vi "Main.vi"() -> ()   [LabVIEW 2017]
uses:
  <vilib>/Utility/error.llb/DialogType.ctl
  <vilib>/Instr/_visa.llb/VISA Configure Serial Port (Serial Instr).vi
panel:
  in  "RUN":bool
  out "Error Messages":string
  in  "Path":path
  in  "Port 2":refnum<visa-resource-name>
  in  "Port 1":refnum<visa-resource-name>
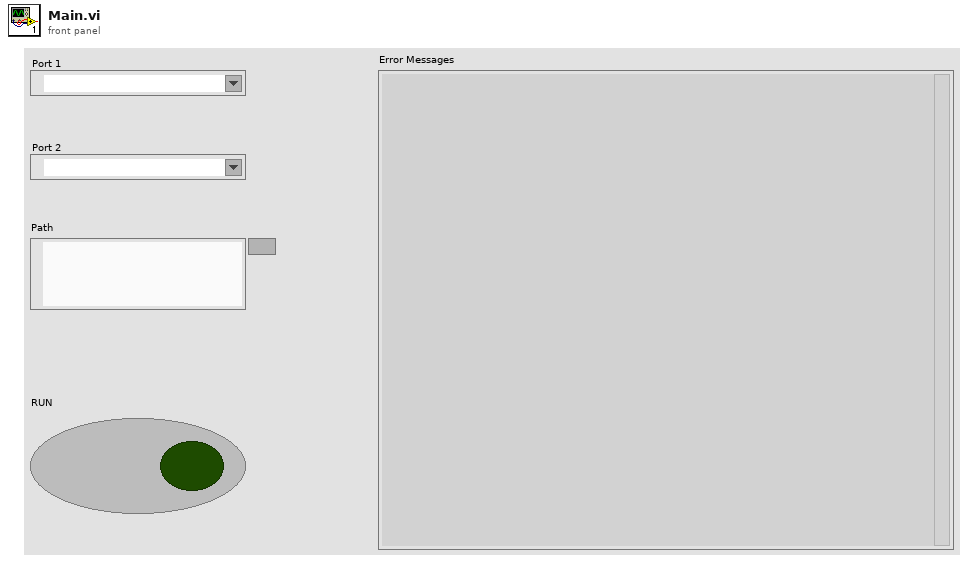
[diagram p1: front panel]
types:
  T1 = cluster{"Port":i8, "Time":timestamp, "Message":string}
  T2 = enum16{"open", "replace", "create", "open or create", "replace or create", "replace or create with confirmation"}
  T3 = typedef "LVDateTimeRec.ctl" = cluster{"fractional second":dbl, "second":i32, "minute":i32, "hour":i32, "day of month":i32, "month":i32, "year":i32, "day of week":i32, "day of year":i32, "DST":i32}
  T4 = typedef "DialogType.ctl" = u16
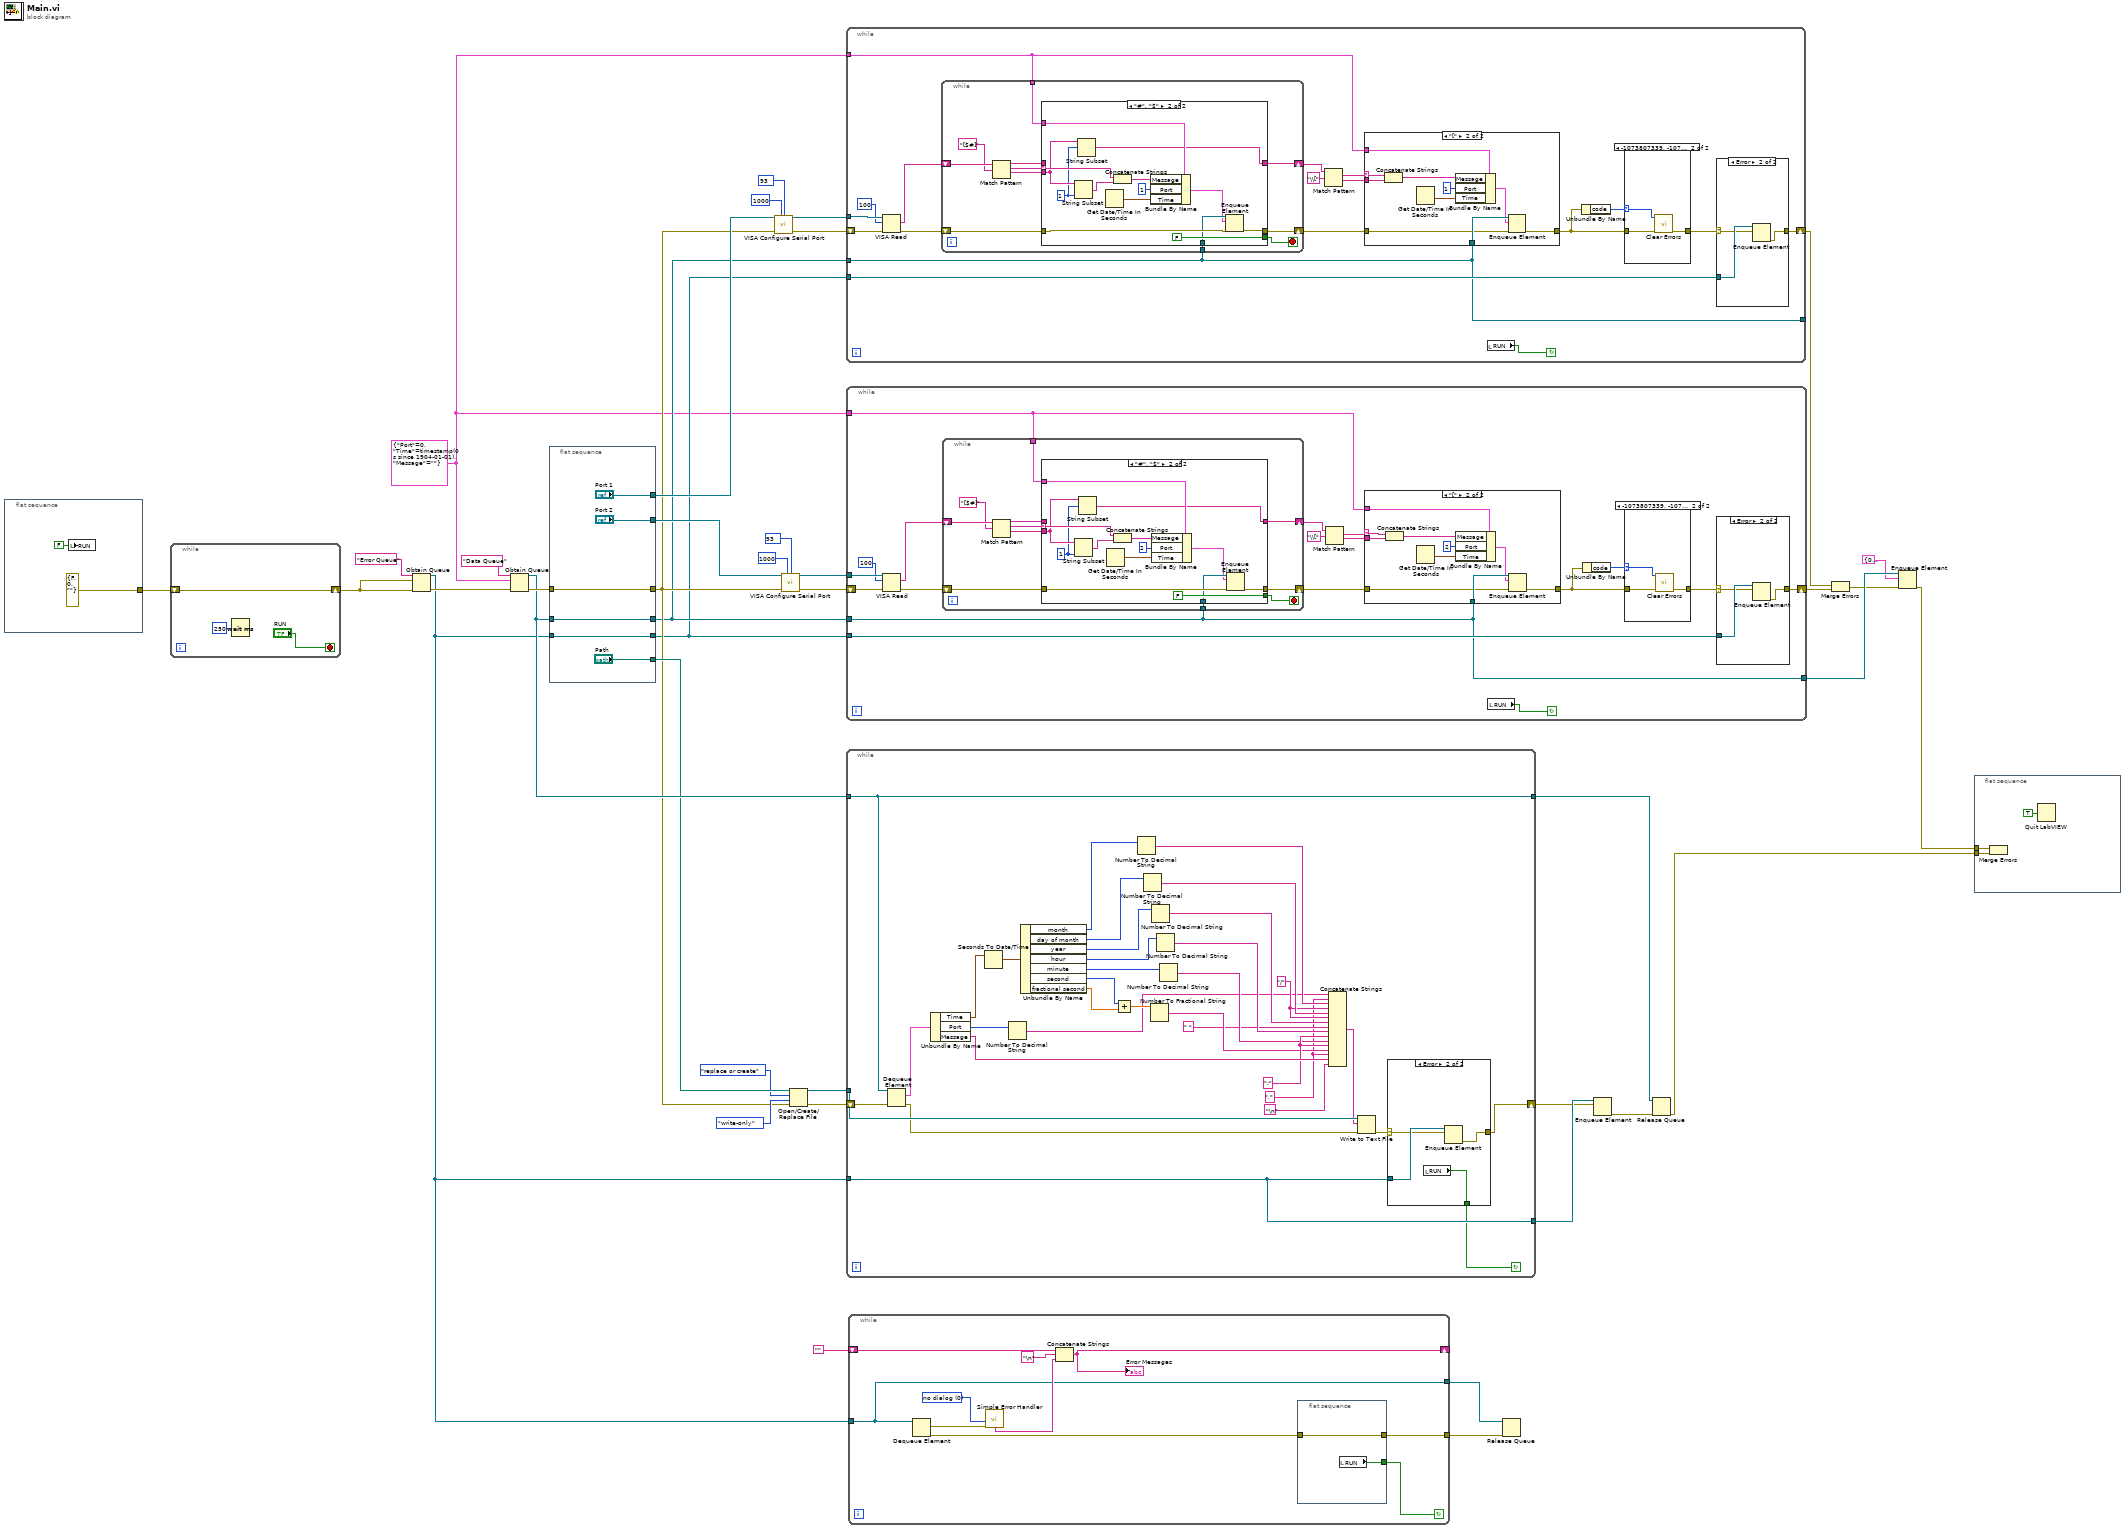
[diagram p0: block diagram]
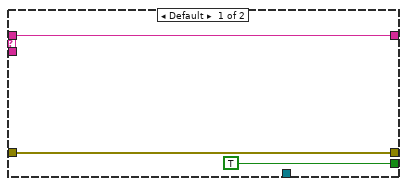
[diagram p2: hidden frame]
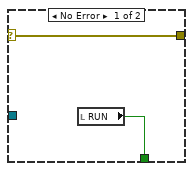
[diagram p6: hidden frame]
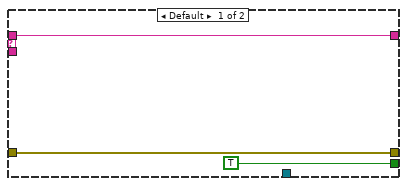
[diagram p7: hidden frame]
diagram:
  w7 = T1 {"Port"=0, "Time"=timestamp(0 s since 1904-01-01), "Message"=""}
  n1 = flat-sequence {
    tunnel: [errorcluster {"status"=FALSE, "code"=0, "source"=""} ("error constant")] -> w41
    frame #0 {
      n2 = local write "RUN"(FALSE ("RUN")) -> ()
    }
  }
  n3 = while {
    shift-right: [w46] -> w40
    shift-left: w41 -> [w46]
    stop <- "RUN" stop-if-true
    n4 = Wait (ms)(milliseconds to wait=u32 250) -> ()  [unwired: 1 out]
  }
  n5 = Obtain Queue(name (unnamed)="Error Queue", element data type=w40, error in (no error)=w40) -> (queue out=w20:refnum<queue>, error out=w38:errorcluster)  [unwired: 2 in, 1 out]
  n6 = Obtain Queue(name (unnamed)="Data Queue", element data type=w7, error in (no error)=w38) -> (queue out=w31:refnum<queue>, error out=w36:errorcluster)  [unwired: 2 in, 1 out]
  n7 = flat-sequence {
    tunnel: w31 -> [w52]
    tunnel: w36 -> [w51]
    tunnel: w20 -> [w50]
    tunnel: [w52] -> w9
    tunnel: [w51] -> w10
    tunnel: [w50] -> w8
    tunnel: ["Port 1"] -> w11
    tunnel: ["Port 2"] -> w12
    tunnel: ["Path"] -> w29
    frame #0 {
    }
  }
  n8 = call-poly "VISA Configure Serial Port"("VISA resource name"=w11, "timeout (10sec)"=u32 1000, "termination char\n(0xA = '\\n' = LF)"=u8 93 ("termination char\n(0xA = '\\n' = LF)"), "error in (no error)"=w10) -> ("VISA resource name out"=w14:refnum<visa-resource-name>, "error out"=w13:errorcluster)  [unwired: 10 in]
  n9 = call-poly "VISA Configure Serial Port"("VISA resource name"=w12, "timeout (10sec)"=u32 1000, "termination char\n(0xA = '\\n' = LF)"=u8 93 ("termination char\n(0xA = '\\n' = LF)"), "error in (no error)"=w10) -> ("VISA resource name out"=w33:refnum<visa-resource-name>, "error out"=w32:errorcluster)  [unwired: 10 in]
  n10 = Open/Create/Replace File(file path (use dialog)=w29, error in=w10, operation (0:open)=T2."replace or create", access (0:read/write)=enum16{"read/write", "read-only", "write-only"}."write-only") -> (refnum out=w30:refnum<file>, error out=w26:errorcluster)  [unwired: 2 in, 1 out]
  n11 = while {
    tunnel: w14 -> [w70]
    tunnel: w7 -> [w55]
    tunnel: w9 -> [w54]
    tunnel: w8 -> [w65]
    shift-right: [w64] -> w5
    shift-left: w13 -> [w69]
    tunnel: [w54] -> _
    stop <- w63 continue-if-true
    n12 = VISA Read(VISA resource name=w70, byte count=u32 100, error in (no error)=w69) -> (read buffer=w58:string, error out=w56:errorcluster)  [unwired: 2 out]
    n13 = while {
      shift-right: [w75] -> w57
      shift-left: w58 -> [w81]
      shift-right: [w74] -> w53
      shift-left: w56 -> [w76]
      tunnel: w55 -> [w72]
      tunnel: w54 -> [w71]
      stop <- w73 stop-if-true
      n14 = Match Pattern(string=w81, regular expression="[$#]") -> (before substring=w78:string, match substring=w79:string, after substring=w77:string)  [unwired: 1 in, 1 out]
      n15 = case shown="\"#\", \"$\"" w79 {
        selector: w79 -> [_ w97]
        tunnel: w78 -> [w84 _]
        tunnel: w77 -> [_ w89]
        tunnel: w76 -> [w83 w94]
        tunnel: [w84 w87] -> w75
        tunnel: [w83 w95] -> w74
        tunnel: [TRUE FALSE] -> w73
        tunnel: w72 -> [_ w92]
        tunnel: w71 -> [_ w93]
        frame Default {
        }
        frame "#", "$" {
          w88 = 1 ("length (rest)")
          n16 = String Subset(string=w89, length (rest)=w88) -> (substring=w96:string)  [unwired: 1 in]
          n17 = String Subset(string=w89, offset (0)=w88) -> (substring=w87:string)  [unwired: 1 in]
          n18 = Get Date/Time In Seconds() -> (seconds since 1Jan1904=w85:timestamp)
          n19 = Concatenate Strings(w97, w96) -> (w90:string)
          n20 = Bundle By Name(cluster=w92, "Message"=w90, "Port"=i8 1, "Time"=w85) -> (w91:T1)
          n21 = Enqueue Element(queue=w93, element=w91, error in (no error)=w94) -> (error out=w95:errorcluster)  [unwired: 1 in, 2 out]
        }
      }
    }
    n22 = Match Pattern(string=w57, regular expression="\\[") -> (match substring=w67:string, after substring=w66:string)  [unwired: 1 in, 2 out]
    n23 = case shown="\"[\"" w67 {
      selector: w67 -> [_ w116]
      tunnel: w66 -> [_ w117]
      tunnel: w55 -> [_ w115]
      tunnel: w53 -> [w107 w110]
      tunnel: w54 -> [_ w111]
      tunnel: [w107 w108] -> w59
      frame Default {
      }
      frame "[" {
        n24 = Concatenate Strings(w116, w117) -> (w114:string)
        n25 = Get Date/Time In Seconds() -> (seconds since 1Jan1904=w112:timestamp)
        n26 = Bundle By Name(cluster=w115, "Message"=w114, "Port"=i8 1, "Time"=w112) -> (w109:T1)
        n27 = Enqueue Element(queue=w111, element=w109, error in (no error)=w110) -> (error out=w108:errorcluster)  [unwired: 1 in, 2 out]
      }
    }
    n28 = local read "RUN"() -> (w63:bool)
    n29 = Unbundle By Name(w59) -> ("code"=w61:i32)
    n30 = case shown="-1073807339, -1073807298, -1073807253" w61 {
      selector: w61 -> [_ w102]
      tunnel: [w99 w100] -> w60
      tunnel: w59 -> [w99 w101]
      frame Default {
      }
      frame -1073807339, -1073807298, -1073807253 {
        n31 = call <vilib>:"Clear Errors.vi"("error in (no error)"=w101, "specific error code to clear (0: all)"=w102) -> ("error out"=w100:errorcluster)  [unwired: 4 in, 1 out]
      }
    }
    n32 = case shown="Error" w60 {
      selector: w60 -> [w103 w105]
      tunnel: w65 -> [_ w106]
      tunnel: [w103 w104] -> w64
      frame No Error {
      }
      frame Error {
        n33 = Enqueue Element(queue=w106, element=w105) -> (error out=w104:errorcluster)  [unwired: 2 in, 2 out]
      }
    }
  }
  n34 = while {
    tunnel: w31 -> [w140]
    tunnel: w30 -> [w146]
    tunnel: w20 -> [w141]
    shift-right: [w142] -> w3
    shift-left: w26 -> [w151]
    tunnel: [w141] -> w23
    tunnel: [w140] -> w21
    stop <- w139 continue-if-true
    w120 = "/" ("string")
    w133 = ":" ("string")
    w119 = "," ("string")
    n35 = Dequeue Element(queue=w140, error in (no error)=w151) -> (element=w150:T1, error out=w144:errorcluster)  [unwired: 1 in, 2 out]
    n36 = Unbundle By Name(w150) -> ("Time"=w138:timestamp, "Port"=w149:i8, "Message"=w148:string)
    n37 = Seconds To Date/Time(time stamp (now)=w138) -> (date time rec=w137:T3)  [unwired: 1 in]
    n38 = Number To Decimal String(number=w149) -> (decimal integer string=w118:string)  [unwired: 1 in]
    n39 = Unbundle By Name(w137) -> ("month"=w125:i32, "day of month"=w126:i32, "year"=w127:i32, "hour"=w128:i32, "minute"=w136:i32, "second"=w134:i32, "fractional second"=w135:dbl)
    n40 = Add(x=w134, y=w135) -> (x+y=w130:dbl)
    n41 = Number To Decimal String(number=w125) -> (decimal integer string=w122:string)  [unwired: 1 in]
    n42 = Number To Decimal String(number=w126) -> (decimal integer string=w123:string)  [unwired: 1 in]
    n43 = Number To Fractional String(number=w130) -> (F-format string=w129:string)  [unwired: 3 in]
    n44 = Number To Decimal String(number=w127) -> (decimal integer string=w124:string)  [unwired: 1 in]
    n45 = Number To Decimal String(number=w128) -> (decimal integer string=w132:string)  [unwired: 1 in]
    n46 = Number To Decimal String(number=w136) -> (decimal integer string=w131:string)  [unwired: 1 in]
    n47 = Concatenate Strings(w118, w119, w122, w120, w123, w120, w124, " ", w132, w133, w131, w133, w129, w119, w148, "\n") -> (w145:string)
    n48 = Write to Text File(file (use dialog)=w146, text=w145, error in=w144) -> (error out=w143:errorcluster)  [unwired: 1 in, 2 out]
    n49 = case shown="Error" w143 {
      selector: w143 -> [w153 w156]
      tunnel: w141 -> [_ w157]
      tunnel: [w153 w155] -> w142
      tunnel: [w152 w154] -> w139
      frame No Error {
        n50 = local read "RUN"() -> (w152:bool)
      }
      frame Error {
        n51 = local read "RUN"() -> (w154:bool)
        n52 = Enqueue Element(queue=w157, element=w156) -> (error out=w155:errorcluster)  [unwired: 2 in, 2 out]
      }
    }
  }
  n53 = while {
    tunnel: w33 -> [w175]
    tunnel: w7 -> [w160]
    tunnel: w9 -> [w159]
    tunnel: w8 -> [w170]
    shift-right: [w169] -> w6
    shift-left: w32 -> [w174]
    tunnel: [w159] -> w25
    stop <- w168 continue-if-true
    n54 = VISA Read(VISA resource name=w175, byte count=u32 100, error in (no error)=w174) -> (read buffer=w163:string, error out=w161:errorcluster)  [unwired: 2 out]
    n55 = while {
      shift-right: [w180] -> w162
      shift-left: w163 -> [w186]
      shift-right: [w179] -> w158
      shift-left: w161 -> [w181]
      tunnel: w160 -> [w177]
      tunnel: w159 -> [w176]
      stop <- w178 stop-if-true
      n56 = Match Pattern(string=w186, regular expression="[$#]") -> (before substring=w183:string, match substring=w184:string, after substring=w182:string)  [unwired: 1 in, 1 out]
      n57 = case shown="\"#\", \"$\"" w184 {
        selector: w184 -> [_ w202]
        tunnel: w183 -> [w189 _]
        tunnel: w182 -> [_ w194]
        tunnel: w181 -> [w188 w199]
        tunnel: [w189 w192] -> w180
        tunnel: [w188 w200] -> w179
        tunnel: [TRUE FALSE] -> w178
        tunnel: w177 -> [_ w197]
        tunnel: w176 -> [_ w198]
        frame Default {
        }
        frame "#", "$" {
          w193 = 1 ("length (rest)")
          n58 = String Subset(string=w194, length (rest)=w193) -> (substring=w201:string)  [unwired: 1 in]
          n59 = String Subset(string=w194, offset (0)=w193) -> (substring=w192:string)  [unwired: 1 in]
          n60 = Get Date/Time In Seconds() -> (seconds since 1Jan1904=w190:timestamp)
          n61 = Concatenate Strings(w202, w201) -> (w195:string)
          n62 = Bundle By Name(cluster=w197, "Message"=w195, "Port"=i8 2, "Time"=w190) -> (w196:T1)
          n63 = Enqueue Element(queue=w198, element=w196, error in (no error)=w199) -> (error out=w200:errorcluster)  [unwired: 1 in, 2 out]
        }
      }
    }
    n64 = Match Pattern(string=w162, regular expression="\\[") -> (match substring=w172:string, after substring=w171:string)  [unwired: 1 in, 2 out]
    n65 = case shown="\"[\"" w172 {
      selector: w172 -> [_ w221]
      tunnel: w171 -> [_ w222]
      tunnel: w160 -> [_ w220]
      tunnel: w158 -> [w212 w215]
      tunnel: w159 -> [_ w216]
      tunnel: [w212 w213] -> w164
      frame Default {
      }
      frame "[" {
        n66 = Concatenate Strings(w221, w222) -> (w219:string)
        n67 = Get Date/Time In Seconds() -> (seconds since 1Jan1904=w217:timestamp)
        n68 = Bundle By Name(cluster=w220, "Message"=w219, "Port"=i8 2, "Time"=w217) -> (w214:T1)
        n69 = Enqueue Element(queue=w216, element=w214, error in (no error)=w215) -> (error out=w213:errorcluster)  [unwired: 1 in, 2 out]
      }
    }
    n70 = local read "RUN"() -> (w168:bool)
    n71 = Unbundle By Name(w164) -> ("code"=w166:i32)
    n72 = case shown="-1073807339, -1073807298, -1073807253" w166 {
      selector: w166 -> [_ w207]
      tunnel: [w204 w205] -> w165
      tunnel: w164 -> [w204 w206]
      frame Default {
      }
      frame -1073807339, -1073807298, -1073807253 {
        n73 = call <vilib>:"Clear Errors.vi"("error in (no error)"=w206, "specific error code to clear (0: all)"=w207) -> ("error out"=w205:errorcluster)  [unwired: 4 in, 1 out]
      }
    }
    n74 = case shown="Error" w165 {
      selector: w165 -> [w208 w210]
      tunnel: w170 -> [_ w211]
      tunnel: [w208 w209] -> w169
      frame No Error {
      }
      frame Error {
        n75 = Enqueue Element(queue=w211, element=w210) -> (error out=w209:errorcluster)  [unwired: 2 in, 2 out]
      }
    }
  }
  n76 = while {
    tunnel: w20 -> [w227]
    shift-right: [w226] -> _
    shift-left: "" -> [w231]
    tunnel: [w227] -> w18
    tunnel: [w224] -> w17
    stop <- w228 continue-if-true
    w232 = T4 0 items=["no dialog", "OK message", "continue or stop message", "OK message + warnings", "continue/stop + warnings"] ("type of dialog (OK msg:1)")
    n77 = Dequeue Element(queue=w227) -> (element=w225:errorcluster, error out=w223:errorcluster)  [unwired: 2 in, 2 out]
    n78 = call <vilib>:"Simple Error Handler.vi"("type of dialog (OK msg:1)"=w232, "error in (no error)"=w225) -> ("message"=w230:string)  [unwired: 3 in, 4 out]
    n79 = Concatenate Strings(w231, "\n" ("string"), w230) -> (w226:string)
    "Error Messages" <- w226
    n80 = flat-sequence {
      tunnel: [w234] -> w228
      tunnel: [w233] -> w224
      tunnel: w223 -> [w233]
      frame #0 {
        n81 = local read "RUN"() -> (w234:bool)
      }
    }
  }
  n82 = Release Queue(queue=w18, error in (no error)=w17) -> ()  [unwired: 1 in, 3 out]
  n83 = Enqueue Element(queue=w23, element=w3) -> (error out=w22:errorcluster)  [unwired: 2 in, 2 out]
  n84 = Release Queue(queue=w21, error in (no error)=w22) -> (error out=w1:errorcluster)  [unwired: 1 in, 2 out]
  n85 = Merge Errors(w5, w6) -> (w4:errorcluster)
  n86 = Enqueue Element(queue=w25, element=T1 {"Port"=0, "Time"=timestamp(0 s since 1904-01-01), "Message"=""}, error in (no error)=w4) -> (error out=w2:errorcluster)  [unwired: 1 in, 2 out]
  n87 = flat-sequence {
    tunnel: w2 -> [w237]
    tunnel: w1 -> [w236]
    frame #0 {
      n88 = Merge Errors(w237, w236) -> ()  [unwired: 1 out]
      n89 = Quit LabVIEW(quit? (T)=TRUE) -> ()
    }
  }
